vi "Play sound right wrong.vi"(9 "Audio":bool, 10 "String":string, 11 "Observer choice":string) -> ()   [LabVIEW 2013]
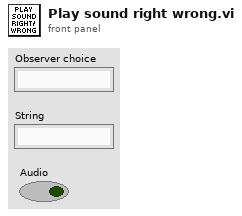
[diagram p1: front panel]
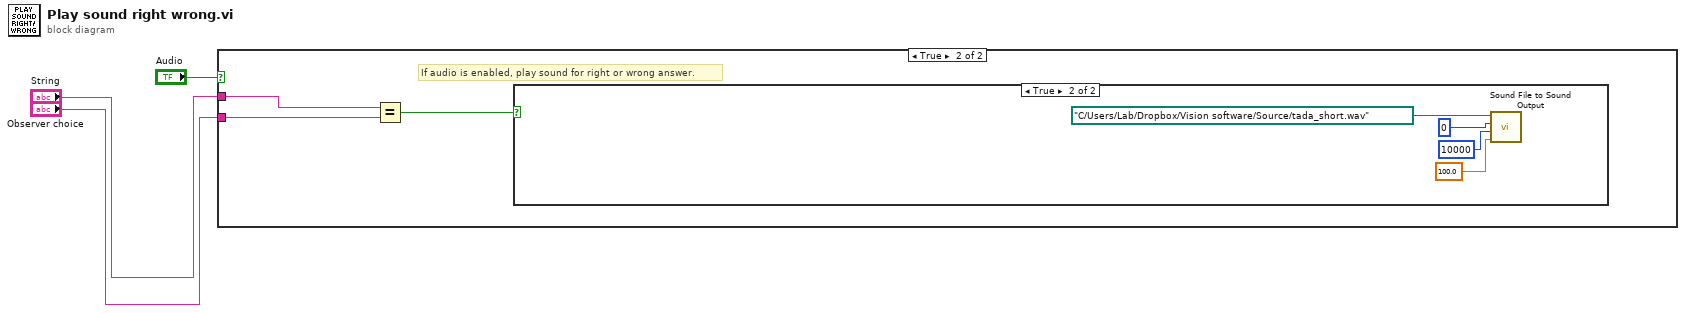
[diagram p0: block diagram]
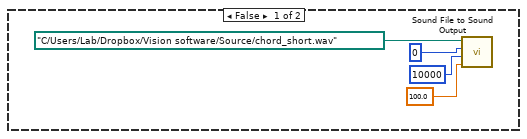
[diagram p3: hidden frame]
diagram:
  n1 = case shown="True" "Audio" {
    tunnel: "String" -> [_ w5]
    tunnel: "Observer choice" -> [_ w4]
    frame False {
    }
    frame True {
      # "If audio is enabled, play sound for right or wrong answer."
      n2 = Equal?(x=w5, y=w4) -> (x = y?=w6:bool)
      n3 = case shown="True" w6 {
        frame False {
          n4 = call "Sound File to Sound Output.vi"("Volume"=100.0, "Number of Samples/Iteration"=10000, "Device ID"=u32 0, "File Path"=path "C:/Users/Lab/Dropbox/Vision software/Source/chord_short.wav") -> ()
        }
        frame True {
          n5 = call "Sound File to Sound Output.vi"("Volume"=100.0, "Number of Samples/Iteration"=10000, "Device ID"=u32 0, "File Path"=path "C:/Users/Lab/Dropbox/Vision software/Source/tada_short.wav") -> ()
        }
      }
    }
  }
